vi "NHMFL Cap Bank Server old.vi"() -> ()   [LabVIEW 2010]
panel:
  out "Active":bool
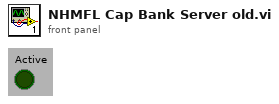
[diagram p1: front panel]
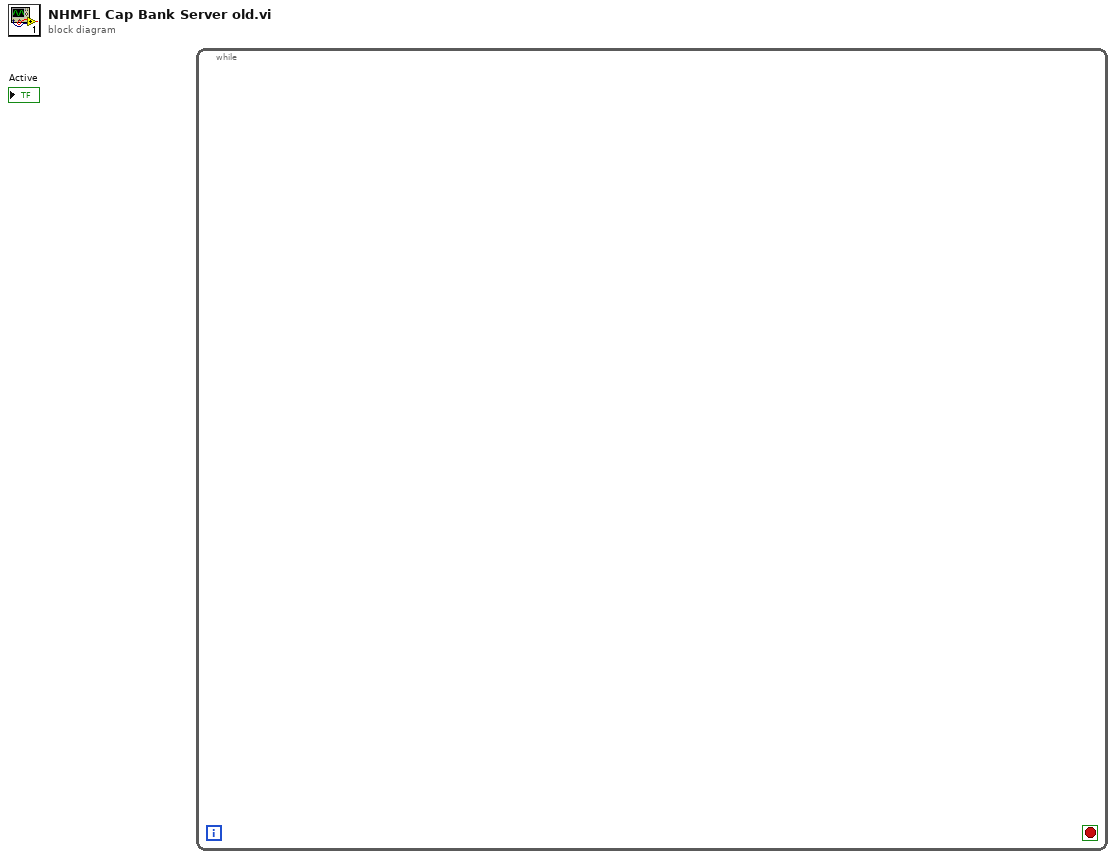
[diagram p0: block diagram]
diagram:
  n1 = while {
    stop <- _ stop-if-true
  }
